vi "Checksum Calculate.vi"(11 "Command in":string) -> (0 "Checksum (byte)":u8 format="%.0x", 1 "Checksum (string)":string, 2 "Command out (with checksum)":string, 3 "Command out (original)":string)   [LabVIEW 2016, in "Samwontech TEMP2xxx.lvlib"]
uses:
  <instrlib>/Samwontech TEMP2xxx/Samwontech TEMP2xxx.lvlib
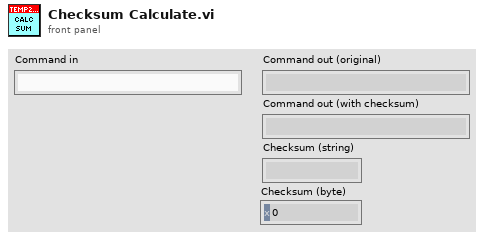
[diagram p1: front panel]
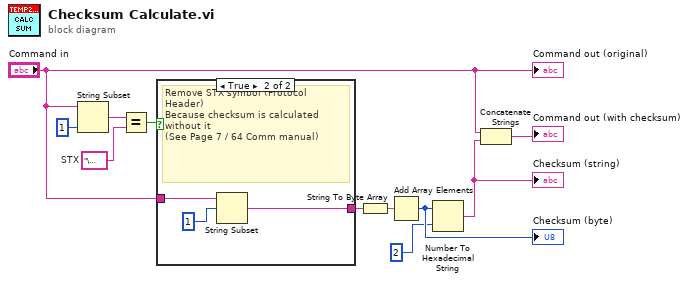
[diagram p0: block diagram]
diagram:
  w9 = "\u0002"  # STX
  n1 = String Subset(string="Command in", length (rest)=1 ("length (rest)")) -> (substring=w10:string)  [unwired: 1 in]
  n2 = Equal?(x=w10, y=w9) -> (x = y?=w8:bool)
  n3 = case shown="True" w8 {
    tunnel: "Command in" -> [w12 w15]
    tunnel: [w12 w13] -> w6
    frame False {
    }
    frame True {
      # "Remove STX symbol (Protocol Header)\nBecause checksum is calculated without it \n(See Page 7 / 64 Comm manual)"
      n4 = String Subset(string=w15, offset (0)=1) -> (substring=w13:string)  [unwired: 1 in]
    }
  }
  n5 = String To Byte Array(string=w6) -> (unsigned byte array=w7:u8[])
  n6 = Add Array Elements(numeric array=w7) -> (sum=w2:u8)
  "Checksum (byte)" <- w2
  n7 = Number To Hexadecimal String(1:i16 2 ("width (-)"), 2:w2) -> (0:w4:string)
  "Checksum (string)" <- w4
  n8 = Concatenate Strings("Command in", w4) -> (→"Command out (with checksum)":string)
  "Command out (original)" <- "Command in"
